vi "Sort_FP_Alarm.vi"(4 "Alarm Status":T2, 6 "Elapsed_SNR_Timer":dbl, 9 "AllAlarms":T4[](array[typedef]), 11 "HDF5_file_refs":T6 {"10HzRefs"."FileRef" format="%.0x"; "10HzRefs"."84Co_dset" format="%.0x"; "10HzRefs"."72Co_dset" format="%.0x"; "AlarmCfg"."84X_CalTonePwr"."ErrsAndWarns" scale=-120.0..-45.0; "AlarmCfg"."72X_CalTonePwr"."ErrsAndWarns" scale=-120.0..-45.0; "AlarmCfg"."84Co_CalTonePwr"."ErrsAndWarns" scale=-120.0..-45.0; "AlarmCfg"."72Co_CalTonePwr"."ErrsAndWarns" scale=-120.0..-45.0; "AlarmCfg"."84CoCalFreq"."ErrsAndWarns" scale=24.9..25.1; "AlarmCfg"."84CoBeacFreq"."ErrsAndWarns" scale=25.5..27.0; "AlarmCfg"."72CoCalFreq"."ErrsAndWarns" scale=24.9..25.1; "AlarmCfg"."72CoBeacFreq"."ErrsAndWarns" scale=25.5..27.0; "AlarmCfg"."ADAM4"."ErrsAndWarns" scale=30.0..52.0; "AlarmCfg"."ADAM3"."ErrsAndWarns" scale=30.0..52.0; "AlarmCfg"."ADAM2"."ErrsAndWarns" scale=30.0..52.0; "AlarmCfg"."ADAM1"."ErrsAndWarns" scale=30.0..52.0; "AlarmCfg"."TE3"."ErrsAndWarns" scale=30.0..52.0; "AlarmCfg"."TE2"."ErrsAndWarns" scale=30.0..52.0; "AlarmCfg"."TE1"."ErrsAndWarns" scale=20.0..52.0; "AlarmCfg"."AI19"."ErrsAndWarns" scale=0.0..60.0; "AlarmCfg"."AI18"."ErrsAndWarns" scale=-10.0..10.0; "AlarmCfg"."AI6"."ErrsAndWarns" scale=0.0..35.0; "AlarmCfg"."AI5"."ErrsAndWarns" scale=0.0..20.0; "AlarmCfg"."AI4"."ErrsAndWarns" scale=0.0..15.0; "AlarmCfg"."AI3"."ErrsAndWarns" scale=0.0..10.0; "AlarmCfg"."AI2"."ErrsAndWarns" scale=0.0..10.0; "AlarmCfg"."TC13"."ErrsAndWarns" scale=-10.0..40.0; "LogData"."NoiseInfo"."HDF5_NoiseInfo"."Sum" format="%^#.1g"; "HDFRefs2"."Complex"."Group_ref" format="%.0x"; "HDFRefs2"."Complex"."QSpect_dset" format="%.0x"; "HDFRefs2"."Complex"."ISpect_dset" format="%.0x"; "HDFRefs2"."Complex"."PwrSpect_dset" format="%.0x"; "HDFRefs2"."Complex"."TImeStamp_dset" format="%.0x"; "HDFRefs2"."ADAM_Refs"."Group_ref" format="%.0x"; "HDFRefs2"."ADAM_Refs"."ADAM_CoPol_dset" format="%.0x"; "HDFRefs2"."ADAM_Refs"."ADAM_XPol_dset" format="%.0x"; "HDFRefs2"."ADAM_Refs"."ADAM_Noise_dset" format="%.0x"; "HDFRefs2"."ADAM_Refs"."ADAM_CalBox_dset" format="%.0x"; "HDFRefs2"."ADAM_Refs"."TimeStamp" format="%.0x"; "HDFRefs2"."Filter_Refs"."Filter_Group_ref" format="%.0x"; "HDFRefs2"."Filter_Refs"."TimeStamp_dset" format="%.0x"; "HDFRefs2"."Filter_Refs"."Filter_dset" format="%.0x"; "HDFRefs2"."AI_Refs"."BlowerPwr_dset" format="%.0x"; "HDFRefs2"."AI_Refs"."ElStdDev_dset" format="%.0x"; "HDFRefs2"."AI_Refs"."AzStdDev_dset" format="%.0x"; "HDFRefs2"."AI_Refs"."AI19_dset" format="%.0x"; "HDFRefs2"."AI_Refs"."AI18_dset" format="%.0x"; "HDFRefs2"."AI_Refs"."AI17_dset" format="%.0x"; "HDFRefs2"."AI_Refs"."AI16_dset" format="%.0x"; "HDFRefs2"."AI_Refs"."AI6_dset" format="%.0x"; "HDFRefs2"."AI_Refs"."AI5_dset" format="%.0x"; "HDFRefs2"."AI_Refs"."AI4_dset" format="%.0x"; "HDFRefs2"."AI_Refs"."AI3_dset" format="%.0x"; "HDFRefs2"."AI_Refs"."AI2_dset" format="%.0x"; "HDFRefs2"."AI_Refs"."AI0_dset" format="%.0x"; "HDFRefs2"."AI_Refs"."AI1_dset" format="%.0x"; "HDFRefs2"."AI_Refs"."TimeString_dset" format="%.0x"; "HDFRefs2"."AI_Refs"."TimeStamp_dset" format="%.0x"; "HDFRefs2"."AI_Refs"."Group_ref" format="%.0x"; "HDFRefs2"."Weath_Refs"."WindDirSTD_dset" format="%.0x"; "HDFRefs2"."Weath_Refs"."WindGusts_dset" format="%.0x"; "HDFRefs2"."Weath_Refs"."RainFall_dset" format="%.0x"; "HDFRefs2"."Weath_Refs"."RainRate_dset" format="%.0x"; "HDFRefs2"."Weath_Refs"."Pressure_dset" format="%.0x"; "HDFRefs2"."Weath_Refs"."Humidity_dset" format="%.0x"; "HDFRefs2"."Weath_Refs"."Temp_dset" format="%.0x"; "HDFRefs2"."Weath_Refs"."WindDir_dset" format="%.0x"; "HDFRefs2"."Weath_Refs"."WindSpd_dset" format="%.0x"; "HDFRefs2"."Weath_Refs"."TimeStamp_dset" format="%.0x"; "HDFRefs2"."Weath_Refs"."Group_ref" format="%.0x"; "HDFRefs2"."Weath_Refs"."TimeString_dset" format="%.0x"; "HDFRefs2"."UPS_Refs_Deprecated"."TimeStamp_dset" format="%.0x"; "HDFRefs2"."UPS_Refs_Deprecated"."TimeString_dset" format="%.0x"; "HDFRefs2"."UPS_Refs_Deprecated"."%_dset" format="%.0x"; "HDFRefs2"."UPS_Refs_Deprecated"."W_dset" format="%.0x"; "HDFRefs2"."UPS_Refs_Deprecated"."Hz_dset" format="%.0x"; "HDFRefs2"."UPS_Refs_Deprecated"."A_dset" format="%.0x"; "HDFRefs2"."UPS_Refs_Deprecated"."V_dset" format="%.0x"; "HDFRefs2"."UPS_Refs_Deprecated"."Group_ref" format="%.0x"; "HDFRefs2"."TE_Refs"."TimeStamp" format="%.0x"; "HDFRefs2"."TE_Refs"."TE_Outp3_dset" format="%.0x"; "HDFRefs2"."TE_Refs"."TE_Temp3_dset" format="%.0x"; "HDFRefs2"."TE_Refs"."TE_Outp2_dset" format="%.0x"; "HDFRefs2"."TE_Refs"."TE_Temp2_dset" format="%.0x"; "HDFRefs2"."TE_Refs"."TE_Outp1_dset" format="%.0x"; "HDFRefs2"."TE_Refs"."TE_Temp1_dset" format="%.0x"; "HDFRefs2"."TE_Refs"."Group_ref" format="%.0x"; "HDFRefs2"."DisdromRefs"."Status_dset_deprecated" format="%.0x"; "HDFRefs2"."DisdromRefs"."Spectrum_dset" format="%.0x"; "HDFRefs2"."DisdromRefs"."SpectGroup_ref" format="%.0x"; "HDFRefs2"."DisdromRefs"."HydromType_dset" format="%.0x"; "HDFRefs2"."DisdromRefs"."UnknownVolum_dset" format="%.0x"; "HDFRefs2"."DisdromRefs"."UnknownParticls_dset" format="%.0x"; "HDFRefs2"."DisdromRefs"."NonHydrVolum_dset" format="%.0x"; "HDFRefs2"."DisdromRefs"."NonHydrParticls_dset" format="%.0x"; "HDFRefs2"."DisdromRefs"."ParticlMinDiam_dset" format="%.0x"; "HDFRefs2"."DisdromRefs"."ParticlMaxSpeed_dset" format="%.0x"; "HDFRefs2"."DisdromRefs"."RadarReflect_dset" format="%.0x"; "HDFRefs2"."DisdromRefs"."Visibility_dset" format="%.0x"; "HDFRefs2"."DisdromRefs"."TotalRain_dset" format="%.0x"; "HDFRefs2"."DisdromRefs"."Solid_dset" format="%.0x"; "HDFRefs2"."DisdromRefs"."Liquid_dset" format="%.0x"; "HDFRefs2"."DisdromRefs"."TotalRainRate_dset" format="%.0x"; "HDFRefs2"."DisdromRefs"."TimeStamp_dset" format="%.0x"; "HDFRefs2"."DisdromRefs"."ParticlMinSpeed_dset" format="%.0x"; "HDFRefs2"."DisdromRefs"."MeasdParticles_dset" format="%.0x"; "HDFRefs2"."DisdromRefs"."MaxDiam_dset" format="%.0x"; "HDFRefs2"."DisdromRefs"."BasicGroup_ref" format="%.0x"; "HDFRefs2"."ValidRefs"."Alarm_Source_dset" format="%.0x"; "HDFRefs2"."ValidRefs"."Time_AlarmChange_dset" format="%.0x"; "HDFRefs2"."ValidRefs"."Time_Valid_dset" format="%.0x"; "HDFRefs2"."ValidRefs"."Alarm_Valid_dset" format="%.0x"; "HDFRefs2"."ValidRefs"."Saturat_dset" format="%.0x"; "HDFRefs2"."ValidRefs"."Group_ref" format="%.0x"; "HDFRefs2"."ValidRefs"."Weath_Valid_dset" format="%.0x"; "HDFRefs2"."ValidRefs"."Disdr_Valid_dset" format="%.0x"; "HDFRefs2"."TC_Refs"."TC13_Tamb_Inter" format="%.0x"; "HDFRefs2"."TC_Refs"."TC12_Gen_Exhaust" format="%.0x"; "HDFRefs2"."TC_Refs"."TC11_HVAC_Cond_Out" format="%.0x"; "HDFRefs2"."TC_Refs"."TC10_HVAC_Cond_In" format="%.0x"; "HDFRefs2"."TC_Refs"."TC9_LP2_Lo" format="%.0x"; "HDFRefs2"."TC_Refs"."TC8_LP2_LoMid" format="%.0x"; "HDFRefs2"."TC_Refs"."TC7_LP2_Mid" format="%.0x"; "HDFRefs2"."TC_Refs"."TC6_LP2_MidHi" format="%.0x"; "HDFRefs2"."TC_Refs"."TC5_LP2_Hi" format="%.0x"; "HDFRefs2"."TC_Refs"."TC4_LP1_Lo" format="%.0x"; "HDFRefs2"."TC_Refs"."TC3_LP1_LoMid" format="%.0x"; "HDFRefs2"."TC_Refs"."TC2_LP1_Mid" format="%.0x"; "HDFRefs2"."TC_Refs"."TC1_LP1_MidHi" format="%.0x"; "HDFRefs2"."TC_Refs"."TC0_LP1_Hi" format="%.0x"; "HDFRefs2"."TC_Refs"."TimeString_dset" format="%.0x"; "HDFRefs2"."TC_Refs"."TimeStamp_dset" format="%.0x"; "HDFRefs2"."TC_Refs"."Group_ref" format="%.0x"; "HDFRefs2"."NoiseRefs"."TimeStamp_df_dset" format="%.0x"; "HDFRefs2"."NoiseRefs"."sum_dset" format="%.0x"; "HDFRefs2"."NoiseRefs"."df_dset" format="%.0x"; "HDFRefs2"."NoiseRefs"."TimeStamp_dset" format="%.0x"; "HDFRefs2"."NoiseRefs"."SumdSpectrum_dset" format="%.0x"; "HDFRefs2"."NoiseRefs"."TimeString_dset" format="%.0x"; "HDFRefs2"."NoiseRefs"."Group_ref" format="%.0x"; "HDFRefs2"."ToneRefs"."Group_ref" format="%.0x"; "HDFRefs2"."ToneRefs"."Cal"."Downshift_dset" format="%.0x"; "HDFRefs2"."ToneRefs"."Cal"."DeltaPhase_dset" format="%.0x"; "HDFRefs2"."ToneRefs"."Cal"."Phase_dset" format="%.0x"; "HDFRefs2"."ToneRefs"."Cal"."SNR_dset" format="%.0x"; "HDFRefs2"."ToneRefs"."Cal"."df_dset" format="%.0x"; "HDFRefs2"."ToneRefs"."Cal"."PeakLoc_dset" format="%.0x"; "HDFRefs2"."ToneRefs"."Cal"."MaxValue_dset" format="%.0x"; "HDFRefs2"."ToneRefs"."Cal"."TImeStamp_dset" format="%.0x"; "HDFRefs2"."ToneRefs"."Cal"."TimeString_dset" format="%.0x"; "HDFRefs2"."ToneRefs"."Beac"."Downshift_dset" format="%.0x"; "HDFRefs2"."ToneRefs"."Beac"."DeltaPhase_dset" format="%.0x"; "HDFRefs2"."ToneRefs"."Beac"."Phase_dset" format="%.0x"; "HDFRefs2"."ToneRefs"."Beac"."SNR_dset" format="%.0x"; "HDFRefs2"."ToneRefs"."Beac"."df_dset" format="%.0x"; "HDFRefs2"."ToneRefs"."Beac"."PeakLoc_dset" format="%.0x"; "HDFRefs2"."ToneRefs"."Beac"."MaxValue_dset" format="%.0x"; "HDFRefs2"."ToneRefs"."Beac"."TImeStamp_dset" format="%.0x"; "HDFRefs2"."ToneRefs"."Beac"."TimeString_dset" format="%.0x"; "HDFRefs2"."ToneRefs"."CalZoom_dSet" format="%.0x"; "HDFRefs2"."ToneRefs"."BeacZoom_dSet" format="%.0x"; "HDFRefs2"."File" format="%.0x"; "HDFRefs1"."Complex"."Group_ref" format="%.0x"; "HDFRefs1"."Complex"."QSpect_dset" format="%.0x"; "HDFRefs1"."Complex"."ISpect_dset" format="%.0x"; "HDFRefs1"."Complex"."PwrSpect_dset" format="%.0x"; "HDFRefs1"."Complex"."TImeStamp_dset" format="%.0x"; "HDFRefs1"."ADAM_Refs"."Group_ref" format="%.0x"; "HDFRefs1"."ADAM_Refs"."ADAM_CoPol_dset" format="%.0x"; "HDFRefs1"."ADAM_Refs"."ADAM_XPol_dset" format="%.0x"; "HDFRefs1"."ADAM_Refs"."ADAM_Noise_dset" format="%.0x"; "HDFRefs1"."ADAM_Refs"."ADAM_CalBox_dset" format="%.0x"; "HDFRefs1"."ADAM_Refs"."TimeStamp" format="%.0x"; "HDFRefs1"."Filter_Refs"."Filter_Group_ref" format="%.0x"; "HDFRefs1"."Filter_Refs"."TimeStamp_dset" format="%.0x"; "HDFRefs1"."Filter_Refs"."Filter_dset" format="%.0x"; "HDFRefs1"."AI_Refs"."BlowerPwr_dset" format="%.0x"; "HDFRefs1"."AI_Refs"."ElStdDev_dset" format="%.0x"; "HDFRefs1"."AI_Refs"."AzStdDev_dset" format="%.0x"; "HDFRefs1"."AI_Refs"."AI19_dset" format="%.0x"; "HDFRefs1"."AI_Refs"."AI18_dset" format="%.0x"; "HDFRefs1"."AI_Refs"."AI17_dset" format="%.0x"; "HDFRefs1"."AI_Refs"."AI16_dset" format="%.0x"; "HDFRefs1"."AI_Refs"."AI6_dset" format="%.0x"; "HDFRefs1"."AI_Refs"."AI5_dset" format="%.0x"; "HDFRefs1"."AI_Refs"."AI4_dset" format="%.0x"; "HDFRefs1"."AI_Refs"."AI3_dset" format="%.0x"; "HDFRefs1"."AI_Refs"."AI2_dset" format="%.0x"; "HDFRefs1"."AI_Refs"."AI0_dset" format="%.0x"; "HDFRefs1"."AI_Refs"."AI1_dset" format="%.0x"; "HDFRefs1"."AI_Refs"."TimeString_dset" format="%.0x"; "HDFRefs1"."AI_Refs"."TimeStamp_dset" format="%.0x"; "HDFRefs1"."AI_Refs"."Group_ref" format="%.0x"; "HDFRefs1"."Weath_Refs"."WindDirSTD_dset" format="%.0x"; "HDFRefs1"."Weath_Refs"."WindGusts_dset" format="%.0x"; "HDFRefs1"."Weath_Refs"."RainFall_dset" format="%.0x"; "HDFRefs1"."Weath_Refs"."RainRate_dset" format="%.0x"; "HDFRefs1"."Weath_Refs"."Pressure_dset" format="%.0x"; "HDFRefs1"."Weath_Refs"."Humidity_dset" format="%.0x"; "HDFRefs1"."Weath_Refs"."Temp_dset" format="%.0x"; "HDFRefs1"."Weath_Refs"."WindDir_dset" format="%.0x"; "HDFRefs1"."Weath_Refs"."WindSpd_dset" format="%.0x"; "HDFRefs1"."Weath_Refs"."TimeStamp_dset" format="%.0x"; "HDFRefs1"."Weath_Refs"."Group_ref" format="%.0x"; "HDFRefs1"."Weath_Refs"."TimeString_dset" format="%.0x"; "HDFRefs1"."UPS_Refs_Deprecated"."TimeStamp_dset" format="%.0x"; "HDFRefs1"."UPS_Refs_Deprecated"."TimeString_dset" format="%.0x"; "HDFRefs1"."UPS_Refs_Deprecated"."%_dset" format="%.0x"; "HDFRefs1"."UPS_Refs_Deprecated"."W_dset" format="%.0x"; "HDFRefs1"."UPS_Refs_Deprecated"."Hz_dset" format="%.0x"; "HDFRefs1"."UPS_Refs_Deprecated"."A_dset" format="%.0x"; "HDFRefs1"."UPS_Refs_Deprecated"."V_dset" format="%.0x"; "HDFRefs1"."UPS_Refs_Deprecated"."Group_ref" format="%.0x"; "HDFRefs1"."TE_Refs"."TimeStamp" format="%.0x"; "HDFRefs1"."TE_Refs"."TE_Outp3_dset" format="%.0x"; "HDFRefs1"."TE_Refs"."TE_Temp3_dset" format="%.0x"; "HDFRefs1"."TE_Refs"."TE_Outp2_dset" format="%.0x"; "HDFRefs1"."TE_Refs"."TE_Temp2_dset" format="%.0x"; "HDFRefs1"."TE_Refs"."TE_Outp1_dset" format="%.0x"; "HDFRefs1"."TE_Refs"."TE_Temp1_dset" format="%.0x"; "HDFRefs1"."TE_Refs"."Group_ref" format="%.0x"; "HDFRefs1"."DisdromRefs"."Status_dset_deprecated" format="%.0x"; "HDFRefs1"."DisdromRefs"."Spectrum_dset" format="%.0x"; "HDFRefs1"."DisdromRefs"."SpectGroup_ref" format="%.0x"; "HDFRefs1"."DisdromRefs"."HydromType_dset" format="%.0x"; "HDFRefs1"."DisdromRefs"."UnknownVolum_dset" format="%.0x"; "HDFRefs1"."DisdromRefs"."UnknownParticls_dset" format="%.0x"; "HDFRefs1"."DisdromRefs"."NonHydrVolum_dset" format="%.0x"; "HDFRefs1"."DisdromRefs"."NonHydrParticls_dset" format="%.0x"; "HDFRefs1"."DisdromRefs"."ParticlMinDiam_dset" format="%.0x"; "HDFRefs1"."DisdromRefs"."ParticlMaxSpeed_dset" format="%.0x"; "HDFRefs1"."DisdromRefs"."RadarReflect_dset" format="%.0x"; "HDFRefs1"."DisdromRefs"."Visibility_dset" format="%.0x"; "HDFRefs1"."DisdromRefs"."TotalRain_dset" format="%.0x"; "HDFRefs1"."DisdromRefs"."Solid_dset" format="%.0x"; "HDFRefs1"."DisdromRefs"."Liquid_dset" format="%.0x"; "HDFRefs1"."DisdromRefs"."TotalRainRate_dset" format="%.0x"; "HDFRefs1"."DisdromRefs"."TimeStamp_dset" format="%.0x"; "HDFRefs1"."DisdromRefs"."ParticlMinSpeed_dset" format="%.0x"; "HDFRefs1"."DisdromRefs"."MeasdParticles_dset" format="%.0x"; "HDFRefs1"."DisdromRefs"."MaxDiam_dset" format="%.0x"; "HDFRefs1"."DisdromRefs"."BasicGroup_ref" format="%.0x"; "HDFRefs1"."ValidRefs"."Alarm_Source_dset" format="%.0x"; "HDFRefs1"."ValidRefs"."Time_AlarmChange_dset" format="%.0x"; "HDFRefs1"."ValidRefs"."Time_Valid_dset" format="%.0x"; "HDFRefs1"."ValidRefs"."Alarm_Valid_dset" format="%.0x"; "HDFRefs1"."ValidRefs"."Saturat_dset" format="%.0x"; "HDFRefs1"."ValidRefs"."Group_ref" format="%.0x"; "HDFRefs1"."ValidRefs"."Weath_Valid_dset" format="%.0x"; "HDFRefs1"."ValidRefs"."Disdr_Valid_dset" format="%.0x"; "HDFRefs1"."TC_Refs"."TC13_Tamb_Inter" format="%.0x"; "HDFRefs1"."TC_Refs"."TC12_Gen_Exhaust" format="%.0x"; "HDFRefs1"."TC_Refs"."TC11_HVAC_Cond_Out" format="%.0x"; "HDFRefs1"."TC_Refs"."TC10_HVAC_Cond_In" format="%.0x"; "HDFRefs1"."TC_Refs"."TC9_LP2_Lo" format="%.0x"; "HDFRefs1"."TC_Refs"."TC8_LP2_LoMid" format="%.0x"; "HDFRefs1"."TC_Refs"."TC7_LP2_Mid" format="%.0x"; "HDFRefs1"."TC_Refs"."TC6_LP2_MidHi" format="%.0x"; "HDFRefs1"."TC_Refs"."TC5_LP2_Hi" format="%.0x"; "HDFRefs1"."TC_Refs"."TC4_LP1_Lo" format="%.0x"; "HDFRefs1"."TC_Refs"."TC3_LP1_LoMid" format="%.0x"; "HDFRefs1"."TC_Refs"."TC2_LP1_Mid" format="%.0x"; "HDFRefs1"."TC_Refs"."TC1_LP1_MidHi" format="%.0x"; "HDFRefs1"."TC_Refs"."TC0_LP1_Hi" format="%.0x"; "HDFRefs1"."TC_Refs"."TimeString_dset" format="%.0x"; "HDFRefs1"."TC_Refs"."TimeStamp_dset" format="%.0x"; "HDFRefs1"."TC_Refs"."Group_ref" format="%.0x"; "HDFRefs1"."NoiseRefs"."TimeStamp_df_dset" format="%.0x"; "HDFRefs1"."NoiseRefs"."sum_dset" format="%.0x"; "HDFRefs1"."NoiseRefs"."df_dset" format="%.0x"; "HDFRefs1"."NoiseRefs"."TimeStamp_dset" format="%.0x"; "HDFRefs1"."NoiseRefs"."SumdSpectrum_dset" format="%.0x"; "HDFRefs1"."NoiseRefs"."TimeString_dset" format="%.0x"; "HDFRefs1"."NoiseRefs"."Group_ref" format="%.0x"; "HDFRefs1"."ToneRefs"."Group_ref" format="%.0x"; "HDFRefs1"."ToneRefs"."Cal"."Downshift_dset" format="%.0x"; "HDFRefs1"."ToneRefs"."Cal"."DeltaPhase_dset" format="%.0x"; "HDFRefs1"."ToneRefs"."Cal"."Phase_dset" format="%.0x"; "HDFRefs1"."ToneRefs"."Cal"."SNR_dset" format="%.0x"; "HDFRefs1"."ToneRefs"."Cal"."df_dset" format="%.0x"; "HDFRefs1"."ToneRefs"."Cal"."PeakLoc_dset" format="%.0x"; "HDFRefs1"."ToneRefs"."Cal"."MaxValue_dset" format="%.0x"; "HDFRefs1"."ToneRefs"."Cal"."TImeStamp_dset" format="%.0x"; "HDFRefs1"."ToneRefs"."Cal"."TimeString_dset" format="%.0x"; "HDFRefs1"."ToneRefs"."Beac"."Downshift_dset" format="%.0x"; "HDFRefs1"."ToneRefs"."Beac"."DeltaPhase_dset" format="%.0x"; "HDFRefs1"."ToneRefs"."Beac"."Phase_dset" format="%.0x"; "HDFRefs1"."ToneRefs"."Beac"."SNR_dset" format="%.0x"; "HDFRefs1"."ToneRefs"."Beac"."df_dset" format="%.0x"; "HDFRefs1"."ToneRefs"."Beac"."PeakLoc_dset" format="%.0x"; "HDFRefs1"."ToneRefs"."Beac"."MaxValue_dset" format="%.0x"; "HDFRefs1"."ToneRefs"."Beac"."TImeStamp_dset" format="%.0x"; "HDFRefs1"."ToneRefs"."Beac"."TimeString_dset" format="%.0x"; "HDFRefs1"."ToneRefs"."CalZoom_dSet" format="%.0x"; "HDFRefs1"."ToneRefs"."BeacZoom_dSet" format="%.0x"; "HDFRefs1"."File" format="%.0x"; "Config"."FP_User"."Deadband" format="%#.0f"}) -> (3 "AlarmDisplay":T1={"Alarms"={"Green"=TRUE, "Rx_Yell"=FALSE, "Cx_Yell"=FALSE, "Red"=FALSE, "Source"=""}, "SerialMeas"={"TE_Air"=0.0, "TE_Bottom"=0.0, "TE_Front"=0.0, "ADAM-Co"=0.0, "ADAM-XPol"=0.0, "ADAM-CalEncl"=0.0, "ADAM-Noise"=0.0}, "AllAlarms"=[], "Elapsed_SNR_Timer"=0.0, "Saturation"={"84"=[], "72"=[]}})   [LabVIEW 2018]
uses:
  LogLoopClust.ctl
  Config_Clust.ctl
  UserConfig.ctl
  PathsCluster.ctl
  FrontPanel_UserConfig.ctl
  Inclinometer_User_Cfg.ctl
  FP_UserTargetConfig.ctl
  FreqShift.ctl
  FPGA_Scale.ctl
  Enums/ScaleMeasure.ctl
  RadioButtons/FilterEnableRadio.ctl
  Enums/TargetNumber.ctl
  HDF5_File_Refs.ctl
  <vilib>/addons/h5labview2/base/hid_t.ctl
  ToneGroupRefsClust.ctl
  HDF5/HDF5_Tone_refs.ctl
  HDF5/HDF5_Noise_refs.ctl
  HDF5/TC_Tone_refs.ctl
  HDF5/HDF5_Validty_refs.ctl
  HDF5/HDF5_Disdrometer_Refs.ctl
  HDF5/HDF5_Health_Refs.ctl
  HDF5/UPS_refs.ctl
  WeatherRefs.ctl
  HDF5/HDF5_AI_refs.ctl
  HDF5/HDF5_Filter_refs.ctl
  HDF5/HDF5_ADAM_Refs.ctl
  HDF5/HDF5_Complex_Refs.ctl
  LogDataClust.ctl
  ToneLogBuffered.ctl
  SaturationMonitorBuffer.ctl
  HDF5/TC_Data_Structure.ctl
  AI_Clust.ctl
  HDF5/HDF5_NoiseInfoClust.ctl
  HDF5/DisdrometerData.ctl
  HDF5/DisdromterSummaryData.ctl
  Disdrometer/Disdrometer_Status_Cluster.ctl
  WeatherDataClust.ctl
  ValidityWeatherClust.ctl
  TE_Data_Clust.ctl
  HDF5/HDF5_ADAM_Data.ctl
  TimeDomainData.ctl
  AlarmSettingsClust.ctl
  AlarmThresh_OneChan.ctl
  ErrorStatus.ctl
  DigOutClust.ctl
  Saturation_Status_Clust.ctl
  HDF5_10HzRefs.ctl
  AlarmDisplay.ctl
  SerialMeasurements_Clust.ctl
types:
  T1 = typedef "AlarmDisplay.ctl" = cluster{"Alarms":T2, "SerialMeas":T3, "AllAlarms":T4[], "Elapsed_SNR_Timer":dbl, "Saturation":T5}
  T2 = typedef "DigOutClust.ctl" = cluster{"Green":bool, "Rx_Yell":bool, "Cx_Yell":bool, "Red":bool, "Source":string}
  T3 = typedef "SerialMeasurements_Clust.ctl" = cluster{"TE_Air":dbl, "TE_Bottom":dbl, "TE_Front":dbl, "ADAM-Co":dbl, "ADAM-XPol":dbl, "ADAM-CalEncl":dbl, "ADAM-Noise":dbl}
  T4 = typedef "ErrorStatus.ctl" = cluster{"RX?":bool, "Warn":bool, "Error":bool, "Enabl":bool, "Source":string}
  T5 = typedef "Saturation_Status_Clust.ctl" = cluster{"84":bool[], "72":bool[]}
  T6 = typedef "LogLoopClust.ctl" = cluster{"base path":path, "PathNow1":path, "PathNow2":path, "DateNow":string, "NAS path":path, "LogFiltStage":bool, "LogNoise_df_1":bool, "LogNoise_df_2":bool, "LogNoise_df_3":bool, "LogNoise_df_4":bool, "Config":T7, "HDFRefs1":T18, "HDFRefs2":T18, "LogData":T33, "AlarmCfg":T47, "DO":bool[], "AllAlarms":T4[], "Alarm Status":T2, "SaturationStatus":T5, "WeatherStatus":bool[], "10HzRefs":T49}
  T7 = typedef "Config_Clust.ctl" = cluster{"UsrCfg":T8, "FP_User":T10}
  T8 = typedef "UserConfig.ctl" = cluster{"Paths":T9, "SampleRate":dbl}
  T9 = typedef "PathsCluster.ctl" = cluster{"CfgFile":path, "LogFolder":path, "LogFile":path, "NAS path":path, "ThreshFile":path, "RedunFolder":path}
  T10 = typedef "FrontPanel_UserConfig.ctl" = cluster{"#NoiseSums":u32, "Max_df":u32, "AvgAvg":bool, "#Avg":u16, "AutoCenter":bool, "Inclin":T11, "1":T12, "2":T12, "3":T12, "4":T12, "Target to Probe":T17, "SNR_Thresh":dbl, "Paths":T9, "Connex_Location":string, "SimulateFPGA":bool, "Deadband":dbl}
  T11 = typedef "Inclinometer_User_Cfg.ctl" = cluster{"Vmin":dbl, "Vmax":dbl, "Angle_min":dbl, "Angle_max":dbl, "Offset":dbl, "Pos_Neg":bool}
  T12 = typedef "FP_UserTargetConfig.ctl" = cluster{"Cal_":T13, "Beac":T13, "Scale":T14, "Offset":fxp<+/-,16,16>, "Scale_Noise":fxp<+/-,30,30>, "Scale_Step1":fxp<+/-,17,17>, "Scale_In_RT":ext, "ScaleMeas":fxp<+/-,16,1>, "FreqsToRemove":i32[], "Width":i32[], "ScaleMeasEnum":T15, "FilterEnab":T16}
  T13 = typedef "FreqShift.ctl" = cluster{"Fine":dbl, "Coarse_":dbl}
  T14 = typedef "FPGA_Scale.ctl" = cluster{"Step4":fxp<+/-,23,23>, "Step5":fxp<+/-,23,23>, "Step6":fxp<+/-,23,23>, "Step7":fxp<+/-,23,23>}
  T15 = typedef "ScaleMeasure.ctl" = enum16{"1", "10", "50", "42"}
  T16 = typedef "FilterEnableRadio.ctl" = enum32{"None", "Step 1", "Frequency Shift", "Step 4", "Step 5", "Step 6", "Step 7"}
  T17 = typedef "TargetNumber.ctl" = enum16{"1", "2", "3", "4"}
  T18 = typedef "HDF5_File_Refs.ctl" = cluster{"File":T19, "ToneRefs":T20[], "NoiseRefs":T22[], "TC_Refs":T23, "ValidRefs":T24, "DisdromRefs":T25, "TE_Refs":T26, "UPS_Refs_Deprecated":T27, "Weath_Refs":T28, "AI_Refs":T29, "Filter_Refs":T30, "ADAM_Refs":T31, "Complex":T32[]}
  T19 = typedef "hid_t.ctl" = i32
  T20 = typedef "ToneGroupRefsClust.ctl" = cluster{"Group_ref":T19, "Cal":T21, "Beac":T21, "CalZoom_dSet":T19, "BeacZoom_dSet":T19}
  T21 = typedef "HDF5_Tone_refs.ctl" = cluster{"TimeString_dset":T19, "TImeStamp_dset":T19, "SNR_dset":T19, "MaxValue_dset":T19, "PeakLoc_dset":T19, "df_dset":T19, "Phase_dset":T19, "DeltaPhase_dset":T19, "Downshift_dset":T19}
  T22 = typedef "HDF5_Noise_refs.ctl" = cluster{"Group_ref":T19, "TimeString_dset":T19, "TimeStamp_dset":T19, "TimeStamp_df_dset":T19, "df_dset":T19, "sum_dset":T19, "SumdSpectrum_dset":T19}
  T23 = typedef "TC_Tone_refs.ctl" = cluster{"Group_ref":T19, "TimeString_dset":T19, "TimeStamp_dset":T19, "TC0_LP1_Hi":T19, "TC1_LP1_MidHi":T19, "TC2_LP1_Mid":T19, "TC3_LP1_LoMid":T19, "TC4_LP1_Lo":T19, "TC5_LP2_Hi":T19, "TC6_LP2_MidHi":T19, "TC7_LP2_Mid":T19, "TC8_LP2_LoMid":T19, "TC9_LP2_Lo":T19, "TC10_HVAC_Cond_In":T19, "TC11_HVAC_Cond_Out":T19, "TC12_Gen_Exhaust":T19, "TC13_Tamb_Inter":T19}
  T24 = typedef "HDF5_Validty_refs.ctl" = cluster{"Group_ref":T19, "Weath_Valid_dset":T19, "Disdr_Valid_dset":T19, "Saturat_dset":T19, "Alarm_Valid_dset":T19, "Time_Valid_dset":T19, "Time_AlarmChange_dset":T19, "Alarm_Source_dset":T19}
  T25 = typedef "HDF5_Disdrometer_Refs.ctl" = cluster{"BasicGroup_ref":T19, "TimeStamp_dset":T19, "TotalRainRate_dset":T19, "Liquid_dset":T19, "Solid_dset":T19, "TotalRain_dset":T19, "Visibility_dset":T19, "RadarReflect_dset":T19, "MaxDiam_dset":T19, "MeasdParticles_dset":T19, "ParticlMinSpeed_dset":T19, "ParticlMaxSpeed_dset":T19, "ParticlMinDiam_dset":T19, "NonHydrParticls_dset":T19, "NonHydrVolum_dset":T19, "UnknownParticls_dset":T19, "UnknownVolum_dset":T19, "HydromType_dset":T19, "SpectGroup_ref":T19, "Spectrum_dset":T19, "Status_dset_deprecated":T19}
  T26 = typedef "HDF5_Health_Refs.ctl" = cluster{"Group_ref":T19, "TE_Temp1_dset":T19, "TE_Outp1_dset":T19, "TE_Temp2_dset":T19, "TE_Outp2_dset":T19, "TE_Temp3_dset":T19, "TE_Outp3_dset":T19, "TimeStamp":T19}
  T27 = typedef "UPS_refs.ctl" = cluster{"Group_ref":T19, "TimeString_dset":T19, "TimeStamp_dset":T19, "V_dset":T19, "A_dset":T19, "Hz_dset":T19, "W_dset":T19, "%_dset":T19}
  T28 = typedef "WeatherRefs.ctl" = cluster{"Group_ref":T19, "TimeString_dset":T19, "TimeStamp_dset ":T19, "WindSpd_dset":T19, "WindGusts_dset":T19, "WindDir_dset":T19, "WindDirSTD_dset":T19, "Temp_dset":T19, "Humidity_dset":T19, "Pressure_dset":T19, "RainRate_dset":T19, "RainFall_dset":T19}
  T29 = typedef "HDF5_AI_refs.ctl" = cluster{"Group_ref":T19, "TimeString_dset":T19, "TimeStamp_dset":T19, "AI0_dset":T19, "AI1_dset":T19, "AI2_dset":T19, "AI3_dset":T19, "AI4_dset":T19, "AI5_dset":T19, "AI6_dset":T19, "AI16_dset":T19, "AI17_dset":T19, "AI18_dset":T19, "AzStdDev_dset":T19, "AI19_dset":T19, "ElStdDev_dset":T19, "BlowerPwr_dset":T19}
  T30 = typedef "HDF5_Filter_refs.ctl" = cluster{"Filter_Group_ref":T19, "TimeStamp_dset":T19, "Filter_dset":T19}
  T31 = typedef "HDF5_ADAM_Refs.ctl" = cluster{"Group_ref":T19, "ADAM_CoPol_dset":T19, "ADAM_XPol_dset":T19, "ADAM_Noise_dset":T19, "ADAM_CalBox_dset":T19, "TimeStamp":T19}
  T32 = typedef "HDF5_Complex_Refs.ctl" = cluster{"Group_ref":T19, "TImeStamp_dset":T19, "PwrSpect_dset":T19, "ISpect_dset":T19, "QSpect_dset":T19}
  T33 = typedef "LogDataClust.ctl" = cluster{"Tone":T34[], "TCData":T36, "AI":T37, "NoiseTrace":cluster{"Target":T17, "NoiseTrace":dbl[]}[], "NoiseInfo":cluster{"Target":T17, "HDF5_NoiseInfo":T38}[], "Disdrom":T39[], "Weath":T42[], "TE":T44, "ADAM":T45, "TimeDomain":T46[]}
  T34 = typedef "ToneLogBuffered.ctl" = cluster{"Count":i32, "CalVal":sgl[], "CalLoc":i32[], "BeacVal":sgl[], "BeacLoc":i32[], "BeacShift":i32[], "Enum":T17, "df":dbl, "PwrSpectr":sgl[][], "ISpectr":sgl[][], "QSpectr":sgl[][], "Time":timestamp[], "SNR":sgl[], "AboveThresh":bool[], "10Hz_PeakVal":dbl[], "Phase":sgl[], "DeltaPhase":dbl[], "Saturat":T35, "10MHz":bool}
  T35 = typedef "SaturationMonitorBuffer.ctl" = cluster{"Meas":bool[], "Stage1":bool[], "Stage4":bool[], "Stage5":bool[], "Stage6":bool[], "Stage7":bool[]}
  T36 = typedef "TC_Data_Structure.ctl" = cluster{"TimeStamp":dbl, "TimeString":string, "TC0_LP1_Hi":dbl, "TC1_LP1_MidHi":dbl, "TC2_LP1_Mid":dbl, "TC3_LP1_LoMid":dbl, "TC4_LP1_Lo":dbl, "TC5_LP2_Hi":dbl, "TC6_LP2_MidHi":dbl, "TC7_LP2_Mid":dbl, "TC8_LP2_LoMid":dbl, "TC9_LP2_Lo":dbl, "TC10_HVAC_Cond_In":dbl, "TC11_HVAC_Cond_Out":dbl, "TC12_Gen_Exhaust":dbl, "TC13_Amb_Inter":dbl, "TC14_Unused":dbl, "TC15_Unused":dbl, "TC16_Unused":dbl, "TC17_Unused":dbl, "TC18_Unused":dbl, "TC19_Unused":dbl, "TC20_Unused":dbl, "TC21_Unused":dbl, "TC22_Unused":dbl, "TC23_Unused":dbl, "TC24_Unused":dbl, "TC25_Unused":dbl, "TC26_Unused":dbl, "TC27_Unused":dbl, "TC28_Unused":dbl, "TC29_Unused":dbl, "TC30_Unused":dbl, "TC31_Unused":dbl}
  T37 = typedef "AI_Clust.ctl" = cluster{"TimeString":string, "Time Stamp":dbl, "AI0_Unused":dbl, "AI1_-5V":dbl, "AI2_+5V":dbl, "AI3_+6V":dbl, "AI4_+12V":dbl, "AI5_+15V":dbl, "AI6_+28V":dbl, "AI7_Unused":dbl, "Ai16_72GHz_CalPower":dbl, "Ai17_84GHz_CalPower":dbl, "Ai18_InclinAz":dbl, "Ai19_InclinEl":dbl, "Ai20_BlowerPwr":dbl, "Ai21_Unused":dbl, "Ai22_Unused":dbl, "Ai23_Unused":dbl, "InclinA_StdDev":dbl, "InclinB_StdDev":dbl, "InclinAz_Unfilt":dbl, "InclinEl_Unfilt":dbl}
  T38 = typedef "HDF5_NoiseInfoClust.ctl" = cluster{"Timestring":string, "Timestamp":dbl, "df":dbl, "Sum":dbl}
  T39 = typedef "DisdrometerData.ctl" = cluster{"Spectrum Data":i16[], "DisdromSummary":T40, "Status":T41}
  T40 = typedef "DisdromterSummaryData.ctl" = cluster{"current time":dbl, "Timestamp":dbl, "Total Rain Rate":dbl, "Liquid Rain Rate":dbl, "Solid Rain Rate":dbl, "Total Rainfall":dbl, "Visibility":dbl, "Radar Reflectivity":dbl, "Max Diameter Hail":dbl, "Measured Particles":i32, "Particle Min Speed":i16, "Particle Max Speed":i16, "Particle Min Diam":i16, "NonHydr Particles":i16, "NonHydr Volume":dbl, "Unkn Particles":i16, "Unkn Volume":dbl, "HydroType":i8}
  T41 = typedef "Disdrometer_Status_Cluster.ctl" = cluster{"Laser":bool, "Signal":bool, "LaserTemp_Analog":bool, "LaserTemp_Digital":bool, "LaserCurrent_Analog":bool, "LaserCurrent_Digital":bool, "SensorSupply":bool, "HeatLaserHead":bool, "HeatReceiverHead":bool, "TempSensor":bool, "HeatSupply":bool, "HeatHousing":bool, "HeatHeads":bool, "HeatCarriers":bool, "OutputLaserPower":bool, "Checksum":bool, "StatusInt":u16}
  T42 = typedef "WeatherDataClust.ctl" = cluster{"TimeString":string, "Timestamp":dbl, "Wind Speed":sgl, "Wind Gusts":sgl, "Wind Dir":sgl, "Wind Dir STD":sgl, "Temperature":sgl, "Humidity":sgl, "Pressure":sgl, "Rain Rate":i16, "Rain Fall":sgl, "Status":T43}
  T43 = typedef "ValidityWeatherClust.ctl" = cluster{"Temp_OutOfBounds":bool, "Temp_IncrSTD":bool, "Temp_Oth":bool, "BarPress_OutOfBounds":bool, "BarPress_IncrSTD":bool, "BarPress_Change":bool, "BarPress_Other":bool, "Humid_OutOfBounds":bool, "Humid_IncrSTD":bool, "Humid_Other":bool, "Wind__Spd_OutOfBounds":bool, "Wind_Dir_OutOfBounds":bool, "RainBuck_OutOfBounds":bool, "RainBuck_Disdrom":bool, "Disdrom_RainBuck":bool, "Placeholder":bool}
  T44 = typedef "TE_Data_Clust.ctl" = cluster{"TimeString":string, "TimeStamp":dbl, "Temp":dbl, "Output":dbl, "Temp 2":dbl, "Output 2":dbl, "Temp 3":dbl, "Output 3":dbl}
  T45 = typedef "HDF5_ADAM_Data.ctl" = cluster{"Timestamp":dbl, "Time string":string, "Fault 1":bool, "Fault 2":bool, "Fault 3":bool, "Fault 4":bool, "Fault 5":bool, "Fault 6":bool, "Value 1":dbl, "Value 2":dbl, "Value 3":dbl, "Value 4":dbl, "Value 5":dbl, "Value 6":dbl}
  T46 = typedef "TimeDomainData.ctl" = cluster{"CalTimeVal":dbl[], "CalTimeCount":u32[], "Enum":T17}
  T47 = typedef "AlarmSettingsClust.ctl" = cluster{"TC13":T48, "AI1":T48, "AI2":T48, "AI3":T48, "AI4":T48, "AI5":T48, "AI6":T48, "AI18":T48, "AI19":T48, "TE1":T48, "TE2":T48, "TE3":T48, "ADAM1":T48, "ADAM2":T48, "ADAM3":T48, "ADAM4":T48, "72CoBeacFreq":T48, "72CoCalFreq":T48, "84CoBeacFreq":T48, "84CoCalFreq":T48, "72Co_CalTonePwr":T48, "72X_CalTonePwr":T48, "84Co_CalTonePwr":T48, "84X_CalTonePwr":T48}
  T48 = typedef "AlarmThresh_OneChan.ctl" = cluster{"Enbl":bool, "ErrsAndWarns":cluster{dbl, dbl, dbl, dbl}}
  T49 = typedef "HDF5_10HzRefs.ctl" = cluster{"72Co_dset":T19, "84Co_dset":T19, "FileRef":T19}
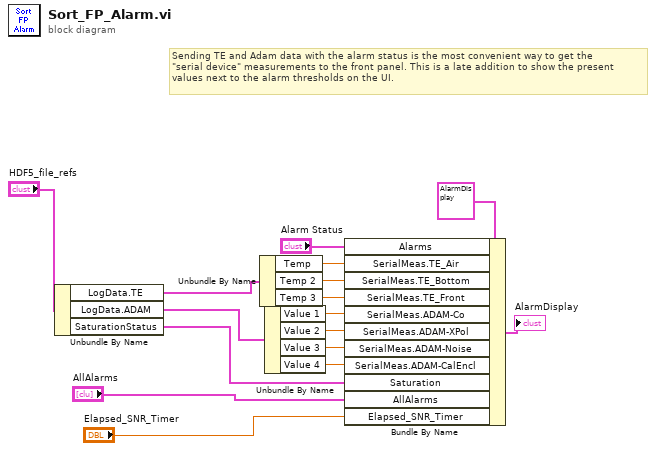
[diagram p0: block diagram]
diagram:
  # "Sending TE and Adam data with the alarm status is the most convenient way to get the \n\"serial device\" measurements to the front panel. This is a late addition to show the present\nvalues next to the alarm thresholds on the UI."
  n1 = Unbundle By Name("HDF5_file_refs") -> ("LogData.TE"=w13:T44, "LogData.ADAM"=w9:T45, "SaturationStatus"=w1:T5)
  n2 = Unbundle By Name(w13) -> ("Temp"=w12:dbl, "Temp 2"=w11:dbl, "Temp 3"=w10:dbl)
  n3 = Unbundle By Name(w9) -> ("Value 1"=w8:dbl, "Value 2"=w7:dbl, "Value 3"=w6:dbl, "Value 4"=w5:dbl)
  n4 = Bundle By Name(cluster=T1 {"Alarms"={"Green"=TRUE, "Rx_Yell"=FALSE, "Cx_Yell"=FALSE, "Red"=FALSE, "Source"=""}, "SerialMeas"={"TE_Air"=0.0, "TE_Bottom"=0.0, "TE_Front"=0.0, "ADAM-Co"=0.0, "ADAM-XPol"=0.0, "ADAM-CalEncl"=0.0, "ADAM-Noise"=0.0}, "AllAlarms"=[], "Elapsed_SNR_Timer"=0.0, "Saturation"={"84"=[], "72"=[]}}, "Alarms"="Alarm Status", "SerialMeas.TE_Air"=w12, "SerialMeas.TE_Bottom"=w11, "SerialMeas.TE_Front"=w10, "SerialMeas.ADAM-Co"=w8, "SerialMeas.ADAM-XPol"=w7, "SerialMeas.ADAM-Noise"=w6, "SerialMeas.ADAM-CalEncl"=w5, "Saturation"=w1, "AllAlarms"="AllAlarms", "Elapsed_SNR_Timer"="Elapsed_SNR_Timer") -> (→"AlarmDisplay":T1)
